vi "Open.vi"(8 "error in (no error)":errorcluster, 11 "LVUnit Test Case in":refnum<class "LVUnit Test Case.lvclass">) -> (0 "error out":errorcluster, 3 "LVUnit Test Case out":refnum<class "LVUnit Test Case.lvclass">)   [LabVIEW 2017, in "LVUnit Test Case.lvclass"]
doc: "Opens the document associated with the test case."
uses:
  LVUnit Test Case.lvclass
  C:/Users/pasca/source/repos/lvunit/Test Case/Test Case.lvclass
  Test Case/Test Case.lvclass/Test Case.ctl
  LVUnit Test Case.lvclass/LVUnit Test Case.ctl
  Test Case/Get Path.vi
  Get JSON Data.vi
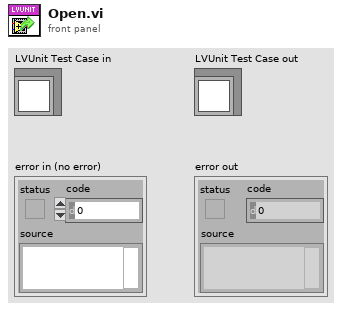
[diagram p1: front panel]
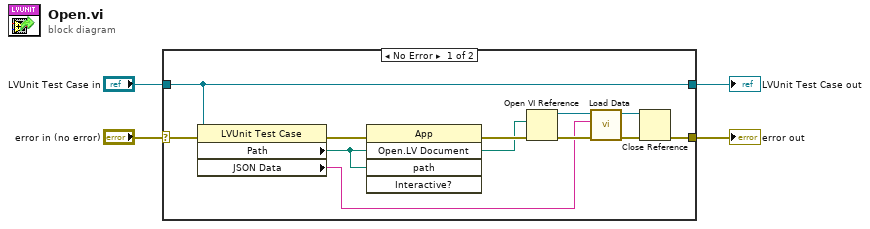
[diagram p0: block diagram]
diagram:
  n1 = case shown="No Error" "error in (no error)" {
    selector: "error in (no error)" -> [w15 w16]
    tunnel: "LVUnit Test Case in" -> [w14 w17]
    tunnel: [w6 w16] -> w2
    tunnel: [w14 w17] -> w1
    frame No Error {
      n2 = property class="LVUnit Test Case"(reference=w14, error in=w15) -> (error out=w9:errorcluster, "Path"=w7:path, "JSON Data"=w10:string)  [unwired: 1 out]
      n3 = invoke class="App" method="Open.LV Document"(error in=w9, "path"=w7) -> (error out=w8:errorcluster)  [unwired: 3 in, 4 out]
      n4 = Open VI Reference(vi path=w7, error in (no error)=w8) -> (vi reference=w11:refnum<vi>, error out=w13:errorcluster)  [unwired: 4 in]
      n5 = call "Load Data.vi"("error in (no error)"=w13, "JSON Data"=w10, "VI Reference"=w11) -> ("error out"=w12:errorcluster, "VI Refnum out"=w5:refnum<vi>)  [unwired: 7 in]
      n6 = Close Reference(reference=w5, error in (no error)=w12) -> (error out=w6:errorcluster)
    }
    frame Error {
    }
  }
  "error out" <- w2
  "LVUnit Test Case out" <- w1
